vi "setSweepTable.vi"(8 "error in (no error)":errorcluster, 9 "Table(s)":variant, 10 "Channel(s)":variant, 11 "Instrument.LockinAPI in":refnum<class "Instrument.LockinAPI.lvclass">) -> (0 "error out":errorcluster, 3 "Instrument.LockinAPI out":refnum<class "Instrument.LockinAPI.lvclass">)   [LabVIEW 2019, in "Instrument.LockinAPI.lvclass"]
doc: "API to set Sweep Waveform"
uses:
  Instrument.LockinAPI.lvclass
  C:/Users/patrick/Documents/GitHub/Instrument-Framework/lvsrc/Instrument/Instrument.lvclass
  Typedefs/API/LockinAPI.Commands--Enum.ctl
  de6fb303-8df8-49ef-b17e-c3f9f1bf9765.vi
  de6fb303-8df8-49ef-b17e-c3f9f1bf9765.vi/8a90de42-1316-4eeb-bb87-fdaf35d44b9d.vi
  de6fb303-8df8-49ef-b17e-c3f9f1bf9765.vi/8a90de42-1316-4eeb-bb87-fdaf35d44b9d.vi/608bd8e6-75ce-4ae9-94dc-a1b4bfe1aa13.vi
  de6fb303-8df8-49ef-b17e-c3f9f1bf9765.vi/8a90de42-1316-4eeb-bb87-fdaf35d44b9d.vi/5dbb763f-d52a-4643-8914-30b67be835a2.vi
  de6fb303-8df8-49ef-b17e-c3f9f1bf9765.vi/8a90de42-1316-4eeb-bb87-fdaf35d44b9d.vi/b1233157-af26-4017-8dfd-887a867efa1e.vi
  <vilib>/JDP Science/JSONtext/Make JSON Array.vi
  de6fb303-8df8-49ef-b17e-c3f9f1bf9765.vi/8a90de42-1316-4eeb-bb87-fdaf35d44b9d.vi/5dbb763f-d52a-4643-8914-30b67be835a2.vi/72826c38-7fda-460d-84d7-86149b90889a.vi
  de6fb303-8df8-49ef-b17e-c3f9f1bf9765.vi/8a90de42-1316-4eeb-bb87-fdaf35d44b9d.vi/b1233157-af26-4017-8dfd-887a867efa1e.vi/47e38901-77d7-4c61-8b0c-bdd41becfc09.vi
  de6fb303-8df8-49ef-b17e-c3f9f1bf9765.vi/8a90de42-1316-4eeb-bb87-fdaf35d44b9d.vi/b1233157-af26-4017-8dfd-887a867efa1e.vi/cfd9f1f3-e76a-4efa-8969-4ff6012f993e.vi
  Instrument/API/Enum to String.vi
  Instrument/Private/Get RC Connection Status.vi
  <vilib>/JDP Science/JSONtext/Variant to JSON Text.vi
  <vilib>/JDP Science/JSONtext/support/Format JSON Array Text.vi
  Instrument/API/Send and Receive.vi
  <vilib>/JDP Science/JSONtext/JSON text to Variant.vi
  <vilib>/JDP Science/JSONtext/LVClass Serializer/JSONtext LVClass Serializer.lvclass
  <vilib>/Utility/Data Type/NI_Data Type.lvlib
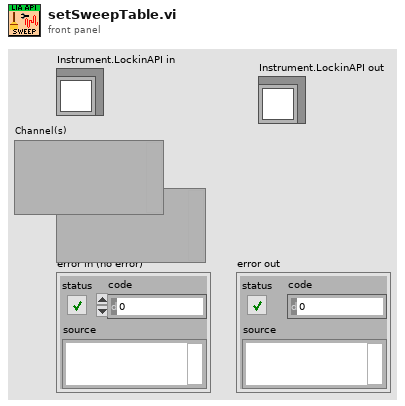
[diagram p1: front panel]
types:
  T1 = cluster{"Sweep Time (s)":dbl, "Initial Wait (s)":dbl, "Return to Start":bool, "Channels":cluster{"Enable?":bool, "Channel":u16, "Start":dbl, "End":dbl, "Pattern":enum16{"Ramp /", "Ramp /\\", "Smooth Ramp _/", "Smooth Ramp _/\\_", "Table"}, "Table":dbl[]}[]}
  T2 = typedef "Instrument.LockinAPI.lvclass/LockinAPI.Commands--Enum.ctl" = enum16{"setAI", "setAO", "setAO_Amplitude", "setAO_DC", "setAO_Frequency", "setAO_Phase", "setAO_Function", "setAO_I+", "setREF", "setREF_Frequency", "setREF_Phase", "setREF_TC", "setREF_Roll-Off", "setDAQ", "setSampling", "setOffset", "setState", "getState", "getAO", "getAI", "getResults", "getSampling", "getAOconfig", "getREFconfig", "setInputGain", "setOutputGain", "getInputGain", "getOutputGain", "setSamplingMode", "getSamplingMode", "setSweep", "setSweepTime", "setSweepTable", "getStatus", "getSweepResults", "getSweepWaveforms", "startSweep", "stopSweep", "setAUX", "getAUX"}
  T3 = cluster{"Enable?":bool, "Channel":u16, "Start":dbl, "End":dbl, "Pattern":enum16{"Ramp /", "Ramp /\\", "Smooth Ramp _/", "Smooth Ramp _/\\_", "Table"}, "Table":dbl[]}[]
  T4 = typedef "NI_Data Type.lvlib/Data Type.ctl" = enum8{"Invalid Type", "Void", "I8", "I16", "I32", "I64", "U8", "U16", "U32", "U64", "Single Float", "Double Float", "Extended Float", "Single Complex", "Double Complex", "Extended Complex", "Enum U8", "Enum U16", "Enum U32", "Enum U64", "Single Float With Unit", "Double Float With Unit", "Extended Float With Unit", "Single Complex with Unit", "Double Complex with Unit", "Extended Complex with Unit", "Boolean", "String", "Path", "Picture", "Tag", "Array", "Cluster", "Variant", "LV Variant", "Waveform", "Timestamp", "Digital Waveform", "Digital Data", "ExpressData", "Refnum", "External Data", "VI", "Poly VI", "LabVIEW Class Instance", "Fixed Point", "Set Collection", "Map Collection"}
  T5 = cluster{"Enable?":bool, "Channel":u16, "Start":dbl, "End":dbl, "Pattern":enum16{"Ramp /", "Ramp /\\", "Smooth Ramp _/", "Smooth Ramp _/\\_", "Table"}, "Table":dbl[]}
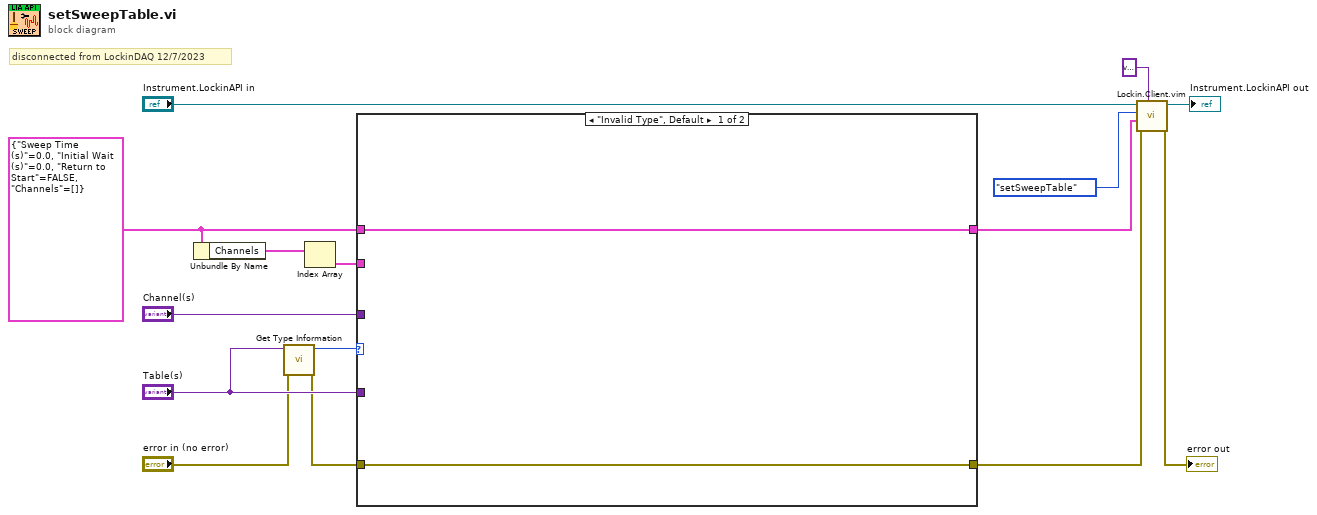
[diagram p0: block diagram]
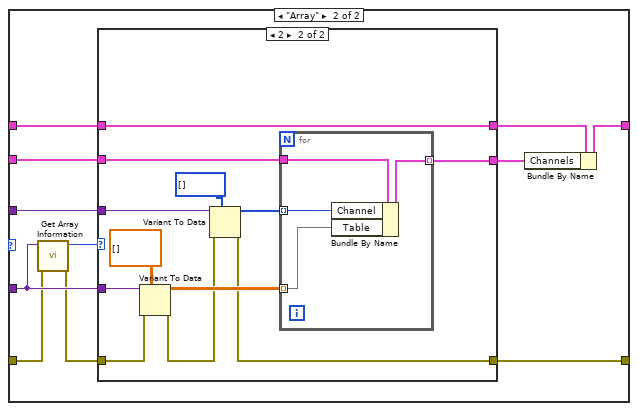
[diagram p2: hidden frame]
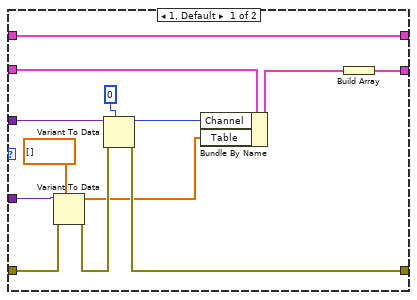
[diagram p3: hidden frame]
diagram:
  w9 = T1 {"Sweep Time (s)"=0.0, "Initial Wait (s)"=0.0, "Return to Start"=FALSE, "Channels"=[]} ("Configure Sweep")
  # "disconnected from LockinDAQ 12/7/2023"
  n1 = Unbundle By Name(w9) -> ("Channels"=w8:T3)
  n2 = call <vilib>:"Get Type Information.vi"("error in (no error)"="error in (no error)", "variant"="Table(s)") -> ("error out"=w3:errorcluster, "type"=w5:T4)  [unwired: 5 in, 3 out]
  n3 = Index Array(array=w8) -> (element=w7:T5)  [unwired: 1 in]
  n4 = case shown="\"Invalid Type\", Default" w5 {
    tunnel: "Channel(s)" -> [_ w28]
    tunnel: w9 -> [w17 w27]
    tunnel: w7 -> [_ w26]
    tunnel: [w17 w20] -> w1
    tunnel: "Table(s)" -> [_ w25]
    tunnel: w3 -> [w16 w23]
    tunnel: [w16 w18] -> w2
    frame "Invalid Type", Default {
    }
    frame "Array" {
      n5 = call <vilib>:"Get Array Information.vi"("error in (no error)"=w23, "variant"=w25) -> ("error out"=w19:errorcluster, "number of dimensions"=w24:i32)  [unwired: 6 in, 2 out]
      n6 = case shown="2" w24 {
        tunnel: w28 -> [w33 w46]
        tunnel: w27 -> [w40 w52]
        tunnel: w26 -> [w41 w53]
        tunnel: [w40 w52] -> w22
        tunnel: [w39 w51] -> w21
        tunnel: w25 -> [w37 w48]
        tunnel: w19 -> [w36 w47]
        tunnel: [w30 w42] -> w18
        frame 1, Default {
          n7 = Variant To Data(error in=w36, type=dbl[] [] ("Pattern"), Variant=w37) -> (data=w29:dbl[], error out=w31:errorcluster)
          n8 = Variant To Data(error in=w31, type=0 ("Channel"), Variant=w33) -> (data=w32:i32, error out=w30:errorcluster)
          n9 = Bundle By Name(cluster=w41, "Channel"=w32, "Table"=w29) -> (w35:T5)
          n10 = Build Array(w35) -> (w39:T3)
        }
        frame 2 {
          n11 = Variant To Data(error in=w47, type=dbl[][] [] ("Pattern"), Variant=w48) -> (data=w49:dbl[][], error out=w43:errorcluster)
          n12 = Variant To Data(error in=w43, type=i32[] [] ("Channel"), Variant=w46) -> (data=w44:i32[], error out=w42:errorcluster)
          n13 = for {
            tunnel: [w54] -> w51 mode=indexing
            tunnel: w49 -> [w57] mode=indexing
            tunnel: w44 -> [w56] mode=indexing
            tunnel: w53 -> [w55]
            n14 = Bundle By Name(cluster=w55, "Channel"=w56, "Table"=w57) -> (w54:T5)
          }
        }
      }
      n15 = Bundle By Name(cluster=w22, "Channels"=w21) -> (w20:T1)
    }
  }
  n16 = call "Lockin.Client.vim"("Data Out type"=variant, "error in (no error)"=w2, "Data"=w1, "Command"=LockinAPI.Commands--Enum."setSweepTable", "Instrument.LockinAPI in"="Instrument.LockinAPI in") -> ("error out"=→"error out":errorcluster, "Instrument.LockinAPI out"=→"Instrument.LockinAPI out":refnum<class "Instrument.LockinAPI.lvclass">)  [unwired: 4 in, 1 out]
